vi "Mexa write D 2.vi"(10 "Array":u8[](array[numeric])=[2, 1, 167, 86]) -> ()   [LabVIEW 2014]
uses:
  <vilib>/rvi/eio/common/nirviEmuTemplateMethod_errors.vi
  <vilib>/eio/EIOMethodNode/EIOMethodNode.xnode
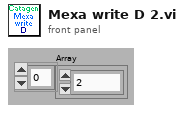
[diagram p1: front panel]
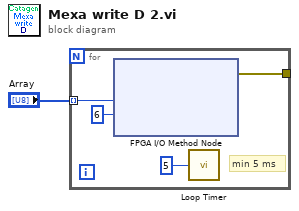
[diagram p0: block diagram]
diagram:
  n1 = for {
    tunnel: [w4] -> _
    tunnel: "Array" -> [w3] mode=indexing
    # "min 5 ms"
    n2 = xnode "FPGA I/O Method Node"("Data"=w3, "Timeout (ms)"=6) -> ("error out"=w4:errorcluster)  [unwired: 2 in, 2 out]
    n3 = call "Loop Timer"("Count(mSec)"=u32 5) -> ()  [unwired: 1 out]
  }
